vi "TIME.vi"(8 "error in":errorcluster, 10 "String":string, 11 "array":path[](array[path])) -> (0 "error out 8":errorcluster)   [LabVIEW 2025]
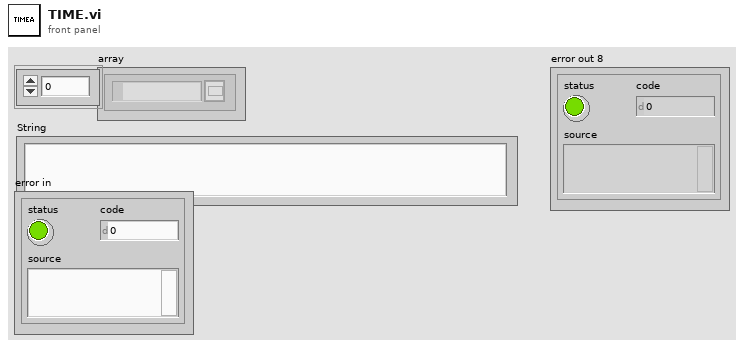
[diagram p1: front panel]
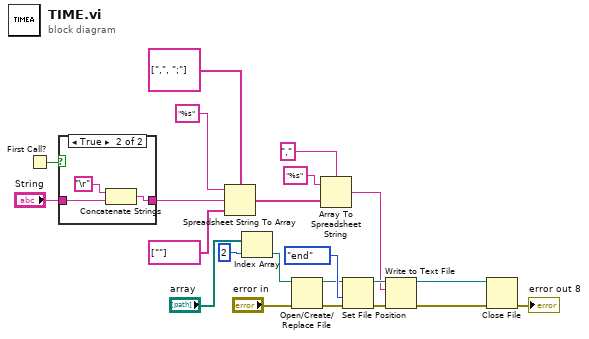
[diagram p0: block diagram]
diagram:
  n1 = First Call?() -> (First Call?: T/F=w7:bool)
  n2 = case shown="True" w7 {
    tunnel: [w23 w25] -> w6
    tunnel: "String" -> [w23 w24]
    frame False {
    }
    frame True {
      n3 = Concatenate Strings("\r", w24) -> (w25:string)
    }
  }
  n4 = Spreadsheet String To Array(delimiter (Tab)=string[] [",", ";"], format string="%s", spreadsheet string=w6, array type (2D Dbl)=string[] [""]) -> (array=w2:string[])
  n5 = Index Array(array="array", index=2 ("index (row)")) -> (element=w12:path)
  n6 = Open/Create/Replace File(file path (use dialog)=w12, error in="error in") -> (refnum out=w13:refnum<file>, error out=w16:errorcluster)  [unwired: 4 in, 1 out]
  n7 = Array To Spreadsheet String(delimiter (Tab)=",", array=w2, 3:"%s" ("format string")) -> (spreadsheet string=w1:string)
  n8 = Set File Position(refnum=w13, from (0:start)=enum16{"start", "end", "current"}."end", error in=w16) -> (refnum out=w14:refnum<file>, error out=w15:errorcluster)  [unwired: 1 in]
  n9 = Write to Text File(file (use dialog)=w14, text=w1, error in=w15) -> (refnum out=w18:refnum<file>, error out=w17:errorcluster)  [unwired: 1 in, 1 out]
  n10 = Close File(refnum=w18, error in=w17) -> (error out=→"error out 8":errorcluster)  [unwired: 1 out]
